vi "创建数据值引用.vi"(8 "error in (no error)":errorcluster caption="错误输入（无错误）", 11 "LS-H600-TCP Client 输入":refnum<class "LS-H600-TCP Client.lvclass">) -> (0 "error out":errorcluster caption="错误输出", 3 "LS-H600-TCP Client 输出":refnum<class "LS-H600-TCP Client.lvclass">)   [LabVIEW 2022 SP3, in "LS-H600-TCP Client.lvlib" / "LS-H600-TCP Client.lvclass"]
uses:
  LS-H600-TCP Client.lvclass
  LS-H600-TCP Client.lvclass/LS-H600-TCP Client.ctl
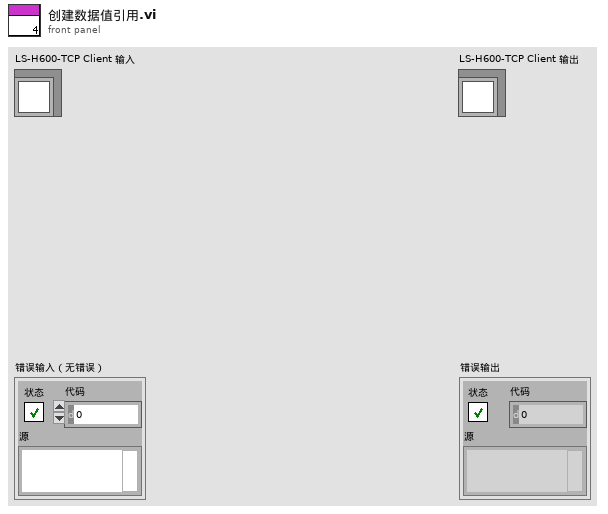
[diagram p1: front panel]
types:
  T1 = cluster{"数据输出":string, "data":cluster{"时间":timestamp, "仪器水深":dbl, "水温":dbl, "流速":dbl, "过水面积":dbl, "瞬时流量":dbl, "累积流量":dbl, "剖面流速":dbl[]}, "连接错误":errorcluster}
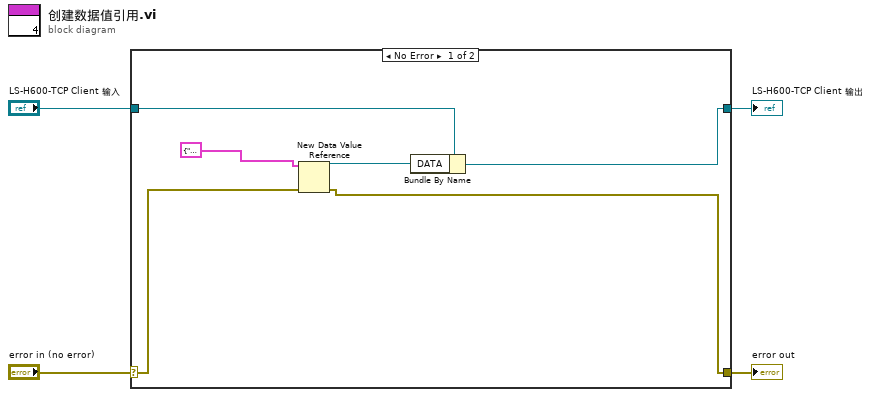
[diagram p0: block diagram]
diagram:
  n1 = case shown="No Error" "error in (no error)" {
    selector: "error in (no error)" -> [w7 w12]
    tunnel: [w6 w12] -> w3
    tunnel: [w8 w11] -> w1
    tunnel: "LS-H600-TCP Client 输入" -> [w10 w11]
    frame No Error {
      n2 = New Data Value Reference(data value=T1 {"数据输出"="", "data"={"时间"=timestamp(0 s since 1904-01-01), "仪器水深"=0.0, "水温"=0.0, "流速"=0.0, "过水面积"=0.0, "瞬时流量"=0.0, "累积流量"=0.0, "剖面流速"=[]}, "连接错误"={"status"=FALSE, "code"=0, "source"=""}} ("DATA"), error in=w7) -> (data value reference=w9:refnum<data-value>, error out=w6:errorcluster)
      n3 = Bundle By Name(cluster=w10, "DATA"=w9) -> (w8:refnum<class "LS-H600-TCP Client.lvclass">)
    }
    frame Error {
    }
  }
  "error out" <- w3
  "LS-H600-TCP Client 输出" <- w1
